vi "S2C_Access_Tables.vi"(8 "Error In":errorcluster) -> (0 "Error Out":errorcluster, 3 "Tables":string[](array[string]))   [LabVIEW 2015]
uses:
  S2C_Access_Globals.vi
  <vilib>/addons/database/NI_Database_API.lvlib
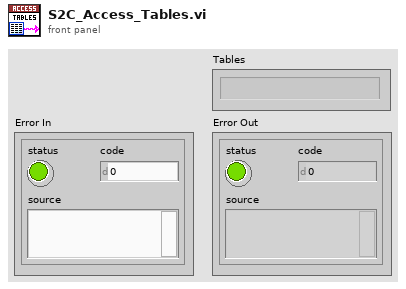
[diagram p1: front panel]
types:
  T1 = typedef "NI_Database_API.lvlib/Conn ObjectReference.ctl" = refnum<k1>
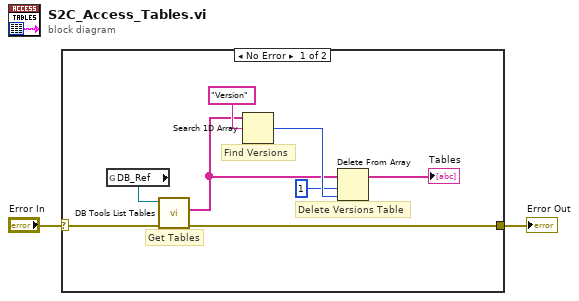
[diagram p0: block diagram]
diagram:
  n1 = case shown="No Error" "Error In" {
    selector: "Error In" -> [w10 w11]
    tunnel: [w8 w11] -> w1
    frame No Error {
      # "Delete Versions Table"
      # "Find Versions"
      # "Get Tables"
      n2 = global read "S2C_Access_Globals.vi" "DB_Ref"() -> (w9:T1)
      n3 = call <vilib>:"DB Tools List Tables.vi"("error in (no error)"=w10, "connection reference"=w9) -> ("error out"=w8:errorcluster, "tables"=w5:string[])  [unwired: 3 in, 1 out]
      n4 = Search 1D Array(1D array=w5, element="Version") -> (index of element=w6:i32)  [unwired: 1 in]
      n5 = Delete From Array(array=w5, length=1, index=w6) -> (array with subset deleted=→"Tables":string[])  [unwired: 1 out]
    }
    frame Error {
    }
  }
  "Error Out" <- w1
